vi "Parse Segments.vi"(8 "error in (no error)":errorcluster, 10 "Proto Path":path, 11 "ProtoParser in":refnum<class "ProtoParser.lvclass">) -> (0 "error out":errorcluster, 2 "Segments":T1[](array[typedef]), 3 "ProtoParser out":refnum<class "ProtoParser.lvclass">)   [LabVIEW 2020, in "LV-Protoc.lvlib" / "ProtoParser.lvclass"]
uses:
  ProtoParser.lvclass
  Segment Type.ctl
  LV-Protoc.lvlib
  Raw Segment.ctl
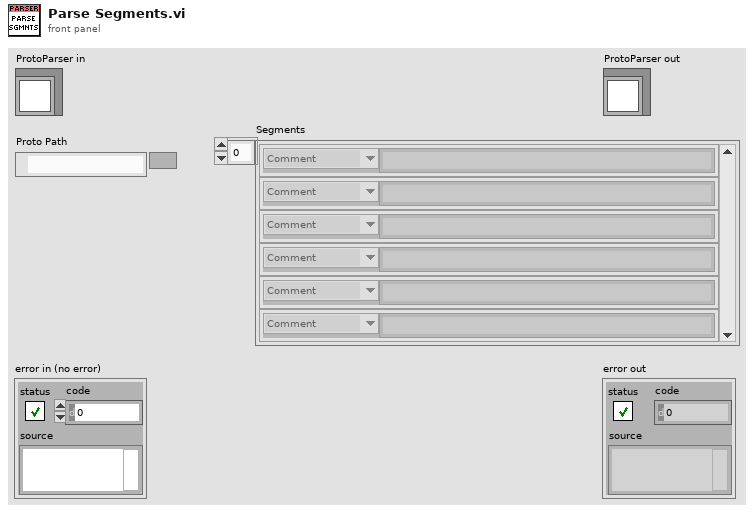
[diagram p1: front panel]
types:
  T1 = typedef "LV-Protoc.lvlib/Raw Segment.ctl" = cluster{"Type":T2, "Text":string}
  T2 = typedef "LV-Protoc.lvlib/Segment Type.ctl" = enum16{"Comment", "Message Open", "Enum Open", "Message Close", "Enum Close", "Field", "Syntax", "Import", "Enum Value", "Package", "Reserved"}
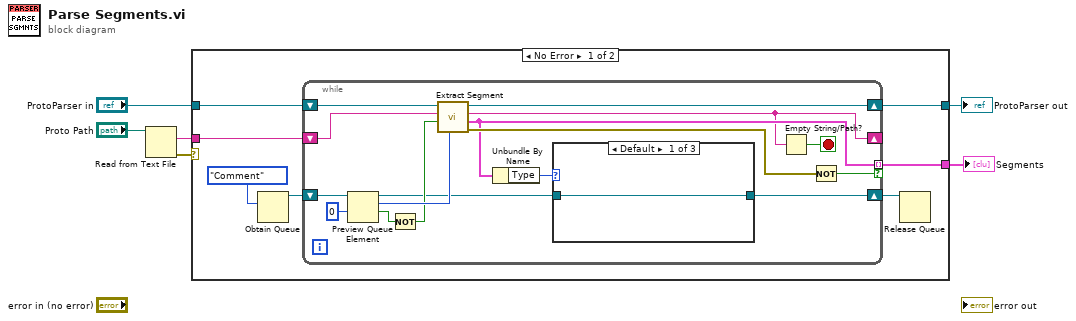
[diagram p0: block diagram]
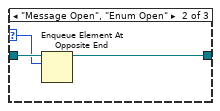
[diagram p2: hidden frame]
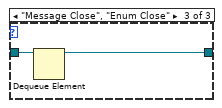
[diagram p3: hidden frame]
diagram:
  n1 = Read from Text File(file (use dialog)="Proto Path") -> (text=w5:string, error out=w4:errorcluster)  [unwired: 3 in, 2 out]
  n2 = case shown="No Error" w4 {
    tunnel: w5 -> [w13 _]
    tunnel: "ProtoParser in" -> [w12 w36]
    tunnel: [w11 w36] -> w2
    tunnel: [w8 _] -> w1
    frame No Error {
      n3 = Obtain Queue(element data type=Segment_Type."Comment" ("Containing Type")) -> (queue out=w9:refnum<queue>)  [unwired: 4 in, 2 out]
      n4 = while {
        shift-right: [w15] -> _
        shift-left: w13 -> [w26]
        shift-right: [w27] -> w11
        shift-left: w12 -> [w28]
        tunnel: [w19] -> w8 mode=indexing if=w25
        shift-right: [w16] -> w7
        shift-left: w9 -> [w24]
        stop <- w14 stop-if-true
        n5 = Preview Queue Element(queue=w24, timeout in ms (-1)=0) -> (queue out=w18:refnum<queue>, element=w23:T2, timed out?=w22:bool)  [unwired: 1 in, 1 out]
        n6 = Not(x=w22) -> (.not. x?=w21:bool)
        n7 = call "Extract Segment.vi"("Containing Type"=w23, "In Type"=w21, "String"=w26, "ProtoParser in"=w28) -> ("error out"=w29:errorcluster, "Segment"=w19:T1, "Remaining"=w15:string, "ProtoParser out"=w27:refnum<class "ProtoParser.lvclass">)  [unwired: 4 in]
        n8 = Unbundle By Name(w19) -> ("Type"=w17:T2)
        n9 = case shown="Default" w17 {
          selector: w17 -> [_ w32 _]
          tunnel: w18 -> [w30 w33 w35]
          tunnel: [w30 w31 w34] -> w16
          frame Default {
          }
          frame "Message Open", "Enum Open" {
            n10 = Enqueue Element At Opposite End(queue=w33, element=w32) -> (queue out=w31:refnum<queue>)  [unwired: 2 in, 2 out]
          }
          frame "Message Close", "Enum Close" {
            n11 = Dequeue Element(queue=w35) -> (queue out=w34:refnum<queue>)  [unwired: 2 in, 3 out]
          }
        }
        n12 = Empty String/Path?(string/path=w15) -> (empty?=w14:bool)
        n13 = Not(x=w29) -> (.not. x?=w25:bool)
      }
      n14 = Release Queue(queue=w7) -> ()  [unwired: 2 in, 3 out]
    }
    frame Error {
    }
  }
  "ProtoParser out" <- w2
  "Segments" <- w1
